vi "PTSequencer.update conditions.vi"(0 "condition in":T1, 1 "data":i8[](array[numeric]), 2 "quality":i32, 3 "Time Stamp":timestamp, 4 "no link":bool) -> (14 "condition out":T1)   [LabVIEW 2014, in "PTSequencer.lvlib"]
uses:
  PTSequencer.lvlib
  PTSequencer.DIM service condition.ctl
  CSCore/CSSystem/CoreDefs/CoreDefs.rawDataType.ctl
  CSCore/CSSystem/CoreLib/CoreLib.byte array 2 string.vi
  CSCore/CSSystem/CoreLib/CoreLib.string 2 byte array.vi
  CSCore/CSSystem/CoreLib/CoreLib.byte array 2 int.vi
  CSCore/CSSystem/CoreLib/CoreLib.int 2 byte array.vi
  CSCore/CSSystem/CoreLib/CoreLib.byte array 2 int array.vi
  CSCore/CSSystem/CoreLib/CoreLib.int array 2 byte array.vi
  CSCore/CSSystem/CoreLib/CoreLib.byte array 2 short.vi
  CSCore/CSSystem/CoreLib/CoreLib.short 2 byte array.vi
  CSCore/CSSystem/CoreLib/CoreLib.byte array 2 short array.vi
  CSCore/CSSystem/CoreLib/CoreLib.short array 2 byte array.vi
  CSCore/CSSystem/CoreLib/CoreLib.byte array 2 double.vi
  CSCore/CSSystem/CoreLib/CoreLib.double 2 byte array.vi
  CSCore/CSSystem/CoreLib/CoreLib.byte array 2 double array.vi
  CSCore/CSSystem/CoreLib/CoreLib.double array 2 byte array.vi
  CSCore/CSSystem/CoreLib/CoreLib.byte array 2 float.vi
  CSCore/CSSystem/CoreLib/CoreLib.float 2 byte array.vi
  CSCore/CSSystem/CoreLib/CoreLib.byte array 2 float array.vi
  CSCore/CSSystem/CoreLib/CoreLib.float array 2 byte array.vi
  CSCore/CSSystem/CoreLib/CoreLib.lvlib
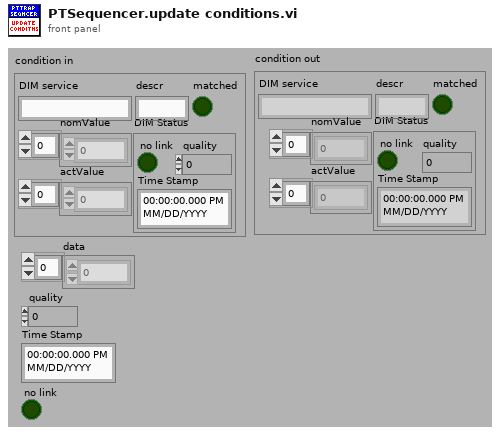
[diagram p1: front panel]
types:
  T1 = typedef "PTSequencer.lvlib/PTSequencer.DIM service condition.ctl" = cluster{"DIM service":string, "descr":string, "nomValue":T2, "actValue":T2, "matched":bool, "DIM Status":cluster{"no link":bool, "quality":i32, "Time Stamp":timestamp}}
  T2 = typedef "CoreDefs.rawDataType.ctl" = i8[]
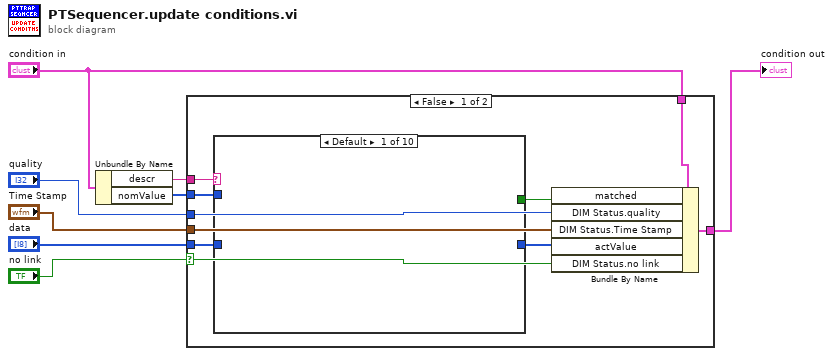
[diagram p0: block diagram]
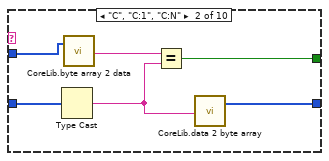
[diagram p2: hidden frame]
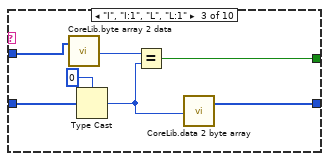
[diagram p3: hidden frame]
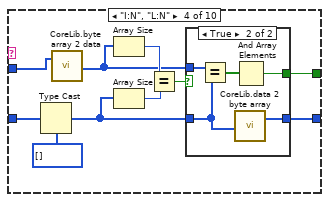
[diagram p4: hidden frame]
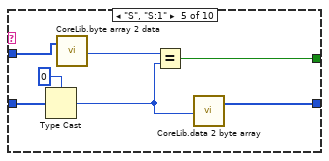
[diagram p6: hidden frame]
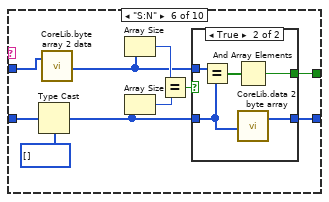
[diagram p7: hidden frame]
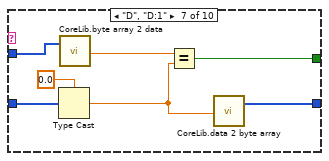
[diagram p9: hidden frame]
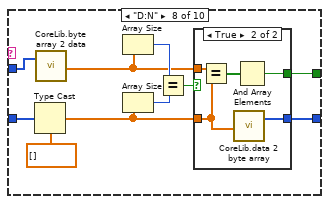
[diagram p10: hidden frame]
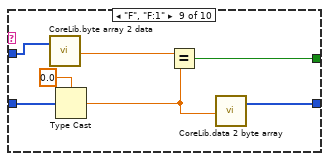
[diagram p12: hidden frame]
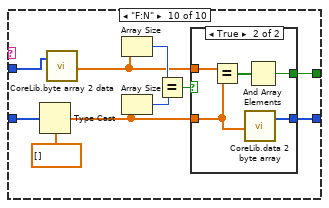
[diagram p13: hidden frame]
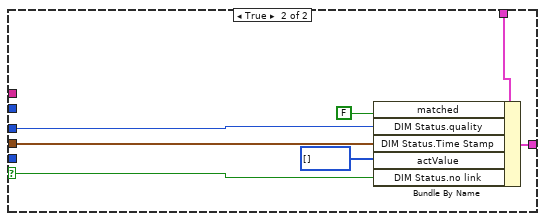
[diagram p15: hidden frame]
diagram:
  n1 = Unbundle By Name("condition in") -> ("descr"=w1:string, "nomValue"=w2:T2)
  n2 = case shown="False" "no link" {
    selector: "no link" -> [w15 w120]
    tunnel: "condition in" -> [w18 w123]
    tunnel: "quality" -> [w17 w122]
    tunnel: "Time Stamp" -> [w16 w121]
    tunnel: "data" -> [w13 _]
    tunnel: [w14 w118] -> w4
    tunnel: w2 -> [w12 _]
    tunnel: w1 -> [w9 _]
    frame False {
      n3 = case shown="Default" w9 {
        tunnel: [_ w24 w31 w40 w54 w63 w77 w86 w100 w109] -> w11
        tunnel: w13 -> [_ w22 w28 w35 w51 w58 w75 w81 w99 w104]
        tunnel: w12 -> [_ w19 w25 w32 w48 w55 w72 w79 w94 w102]
        tunnel: [_ w23 w30 w34 w53 w57 w74 w80 w97 w103] -> w10
        frame Default {
        }
        frame "C", "C:1", "C:N" {
          n4 = Type Cast(x=w22) -> (*(type *) &x=w21:string)  [unwired: 1 in]
          n5 = call-poly "CoreLib.byte array 2 data.vi"("byteArray"=w19) -> ("string"=w20:string)  [unwired: 16 in, 2 out]
          n6 = Equal?(x=w20, y=w21) -> (x = y?=w24:bool)
          n7 = call-poly "CoreLib.data 2 byte array.vi"("string"=w21) -> ("byteArray out"=w23:T2)  [unwired: 18 in]
        }
        frame "I", "I:1", "L", "L:1" {
          n8 = call-poly "CoreLib.byte array 2 data.vi"("byteArray"=w25) -> ("i32"=w26:i32)  [unwired: 16 in, 2 out]
          n9 = Type Cast(type=0, x=w28) -> (*(type *) &x=w29:i32)
          n10 = Equal?(x=w26, y=w29) -> (x = y?=w31:bool)
          n11 = call-poly "CoreLib.data 2 byte array.vi"("i32"=w29) -> ("byteArray out"=w30:T2)  [unwired: 18 in]
        }
        frame "I:N", "L:N" {
          n12 = Type Cast(type=i32[] [], x=w35) -> (*(type *) &x=w36:i32[])
          n13 = call-poly "CoreLib.byte array 2 data.vi"("byteArray"=w32) -> ("[i32]"=w33:i32[])  [unwired: 16 in, 2 out]
          n14 = Array Size(array=w33) -> (size(s)=w38:i32)
          n15 = Array Size(array=w36) -> (size(s)=w39:i32)
          n16 = Equal?(x=w38, y=w39) -> (x = y?=w37:bool)
          n17 = case shown="True" w37 {
            selector: w37 -> [w42 _]
            tunnel: [w42 w46] -> w40
            tunnel: w36 -> [_ w44]
            tunnel: w33 -> [_ w45]
            tunnel: [_ w43] -> w34
            frame False {
            }
            frame True {
              n18 = Equal?(x=w45, y=w44) -> (x = y?=w47:bool[])
              n19 = call-poly "CoreLib.data 2 byte array.vi"("[i32]"=w44) -> ("byteArray out"=w43:T2)  [unwired: 18 in]
              n20 = And Array Elements(Boolean array=w47) -> (logical AND=w46:bool)
            }
          }
        }
        frame "S", "S:1" {
          n21 = Type Cast(type=i16 0, x=w51) -> (*(type *) &x=w52:i16)
          n22 = call-poly "CoreLib.byte array 2 data.vi"("byteArray"=w48) -> ("i16"=w49:i16)  [unwired: 16 in, 2 out]
          n23 = Equal?(x=w49, y=w52) -> (x = y?=w54:bool)
          n24 = call-poly "CoreLib.data 2 byte array.vi"("i16"=w52) -> ("byteArray out"=w53:T2)  [unwired: 18 in]
        }
        frame "S:N" {
          n25 = Type Cast(type=i16[] [], x=w58) -> (*(type *) &x=w59:i16[])
          n26 = call-poly "CoreLib.byte array 2 data.vi"("byteArray"=w55) -> ("[i16]"=w56:i16[])  [unwired: 16 in, 2 out]
          n27 = Array Size(array=w56) -> (size(s)=w62:i32)
          n28 = Array Size(array=w59) -> (size(s)=w61:i32)
          n29 = Equal?(x=w62, y=w61) -> (x = y?=w60:bool)
          n30 = case shown="True" w60 {
            selector: w60 -> [w65 _]
            tunnel: w56 -> [_ w70]
            tunnel: w59 -> [_ w66]
            tunnel: [w65 w68] -> w63
            tunnel: [_ w67] -> w57
            frame False {
            }
            frame True {
              n31 = Equal?(x=w70, y=w66) -> (x = y?=w69:bool[])
              n32 = And Array Elements(Boolean array=w69) -> (logical AND=w68:bool)
              n33 = call-poly "CoreLib.data 2 byte array.vi"("[i16]"=w66) -> ("byteArray out"=w67:T2)  [unwired: 18 in]
            }
          }
        }
        frame "D", "D:1" {
          n34 = Type Cast(type=0.0, x=w75) -> (*(type *) &x=w73:dbl)
          n35 = call-poly "CoreLib.byte array 2 data.vi"("byteArray"=w72) -> ("d64"=w71:dbl)  [unwired: 16 in, 2 out]
          n36 = Equal?(x=w71, y=w73) -> (x = y?=w77:bool)
          n37 = call-poly "CoreLib.data 2 byte array.vi"("f64"=w73) -> ("byteArray out"=w74:T2)  [unwired: 18 in]
        }
        frame "D:N" {
          n38 = Type Cast(type=dbl[] [], x=w81) -> (*(type *) &x=w82:dbl[])
          n39 = call-poly "CoreLib.byte array 2 data.vi"("byteArray"=w79) -> ("[d64]"=w78:dbl[])  [unwired: 16 in, 2 out]
          n40 = Array Size(array=w78) -> (size(s)=w85:i32)
          n41 = Array Size(array=w82) -> (size(s)=w84:i32)
          n42 = Equal?(x=w85, y=w84) -> (x = y?=w83:bool)
          n43 = case shown="True" w83 {
            selector: w83 -> [w88 _]
            tunnel: w78 -> [_ w93]
            tunnel: w82 -> [_ w89]
            tunnel: [w88 w91] -> w86
            tunnel: [_ w90] -> w80
            frame False {
            }
            frame True {
              n44 = Equal?(x=w93, y=w89) -> (x = y?=w92:bool[])
              n45 = call-poly "CoreLib.data 2 byte array.vi"("[d64]"=w89) -> ("byteArray out"=w90:T2)  [unwired: 18 in]
              n46 = And Array Elements(Boolean array=w92) -> (logical AND=w91:bool)
            }
          }
        }
        frame "F", "F:1" {
          n47 = call-poly "CoreLib.byte array 2 data.vi"("byteArray"=w94) -> ("f32"=w95:sgl)  [unwired: 16 in, 2 out]
          n48 = Type Cast(type=sgl 0.0, x=w99) -> (*(type *) &x=w96:sgl)
          n49 = Equal?(x=w95, y=w96) -> (x = y?=w100:bool)
          n50 = call-poly "CoreLib.data 2 byte array.vi"("f32"=w96) -> ("byteArray out"=w97:T2)  [unwired: 18 in]
        }
        frame "F:N" {
          n51 = Type Cast(type=sgl[] [], x=w104) -> (*(type *) &x=w105:sgl[])
          n52 = call-poly "CoreLib.byte array 2 data.vi"("byteArray"=w102) -> ("[f32]"=w101:sgl[])  [unwired: 16 in, 2 out]
          n53 = Array Size(array=w101) -> (size(s)=w106:i32)
          n54 = Array Size(array=w105) -> (size(s)=w108:i32)
          n55 = Equal?(x=w106, y=w108) -> (x = y?=w107:bool)
          n56 = case shown="True" w107 {
            selector: w107 -> [w111 _]
            tunnel: w101 -> [_ w116]
            tunnel: w105 -> [_ w112]
            tunnel: [w111 w114] -> w109
            tunnel: [_ w113] -> w103
            frame False {
            }
            frame True {
              n57 = Equal?(x=w116, y=w112) -> (x = y?=w115:bool[])
              n58 = call-poly "CoreLib.data 2 byte array.vi"("[f32]"=w112) -> ("byteArray out"=w113:T2)  [unwired: 18 in]
              n59 = And Array Elements(Boolean array=w115) -> (logical AND=w114:bool)
            }
          }
        }
      }
      n60 = Bundle By Name(cluster=w18, "matched"=w11, "DIM Status.quality"=w17, "DIM Status.Time Stamp"=w16, "actValue"=w10, "DIM Status.no link"=w15) -> (w14:T1)
    }
    frame True {
      n61 = Bundle By Name(cluster=w123, "matched"=FALSE, "DIM Status.quality"=w122, "DIM Status.Time Stamp"=w121, "actValue"=i8[] [] ("data 2"), "DIM Status.no link"=w120) -> (w118:T1)
    }
  }
  "condition out" <- w4
